vi "Msg.Sequence Number Counter.vi"() -> (0 "SeqNum":i32)   [LabVIEW 2024, in "EQMF.lvlib" / "Queue Utils.lvlib"]
uses:
  Queue Utils.lvlib
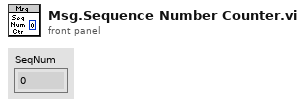
[diagram p1: front panel]
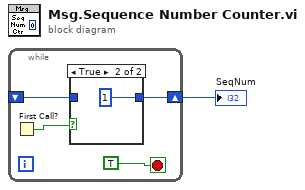
[diagram p0: block diagram]
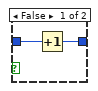
[diagram p2: hidden frame]
diagram:
  n1 = while {
    shift-right: [w2] -> w1
    shift-left: _ -> [w3]
    stop <- TRUE stop-if-true
    n2 = First Call?() -> (First Call?: T/F=w4:bool)
    n3 = case shown="True" w4 {
      tunnel: w3 -> [w6 _]
      tunnel: [w7 1 ("SeqNum")] -> w2
      frame False {
        n4 = Increment(x=w6) -> (x+1=w7:i32)
      }
      frame True {
      }
    }
  }
  "SeqNum" <- w1
